vi "UI - Main UI config.vi"() -> ()   [LabVIEW 2020, in "Configuration.lvclass"]
doc: "Module UI that appears in the Configuration UI.\n____\nPeloton Config 2.0.0.9\nCopyright (c) 2024, Peloton"
uses:
  Configuration.lvclass
  <vilib>/Peloton/Peloton Config/DCFG Framework/Init UI Params--cluster.ctl
  <vilib>/Peloton/Peloton Config/DCFG Framework/Configuration_class/Configuration.lvclass
  <vilib>/Peloton/Peloton Config/DCFG Framework/Stop Argument--cluster.ctl
  <vilib>/Peloton/Peloton Config/DCFG Framework/Send Config to Page Argument--cluster.ctl
  <vilib>/Peloton/Peloton Config/DCFG Framework/Send Stop to Page Argument--cluster.ctl
  C:/Program Files (x86)/National Instruments/LabVIEW 2020/vi.lib/Peloton/Peloton Config/DCFG Framework/Configuration_class/Configuration.lvclass
  <vilib>/Peloton/Peloton Config/DCFG Framework/Configuration_class/Configuration.lvclass/Configuration.ctl
  Configuration--cluster.ctl
  Configuration.lvclass/Configuration.ctl
  Set Configuration.vi
  Get Configuration.vi
  <vilib>/Peloton/Peloton Config/DCFG Framework/Configuration_class/Get Name.vi
  <vilib>/Peloton/Peloton Config/DCFG Framework/Peloton_lib_DCFG Framework.lvlib
panel:
  in  "B":dbl
  in  "a":dbl
  in  "Init UI Params":T1
  # "Define the Default Configuration UI here."
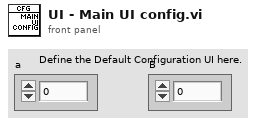
[diagram p1: front panel]
types:
  T1 = typedef "Peloton_lib_DCFG Framework.lvlib/Init UI Params--cluster.ctl" = cluster{"Initial Config":refnum<class "Configuration.lvclass">, "Stop CFG Module":refnum<user-event>, "Send Config to Page":refnum<user-event>, "Send Stop to Page":refnum<user-event>, "Reset Page Defaults":refnum<user-event>}
  T2 = enum32{"Invalid", "Standard", "Closed", "Hidden", "Minimized", "Maximized"}
  T3 = typedef "Configuration.lvclass/Configuration--cluster.ctl" = cluster{"a":dbl, "B":dbl}
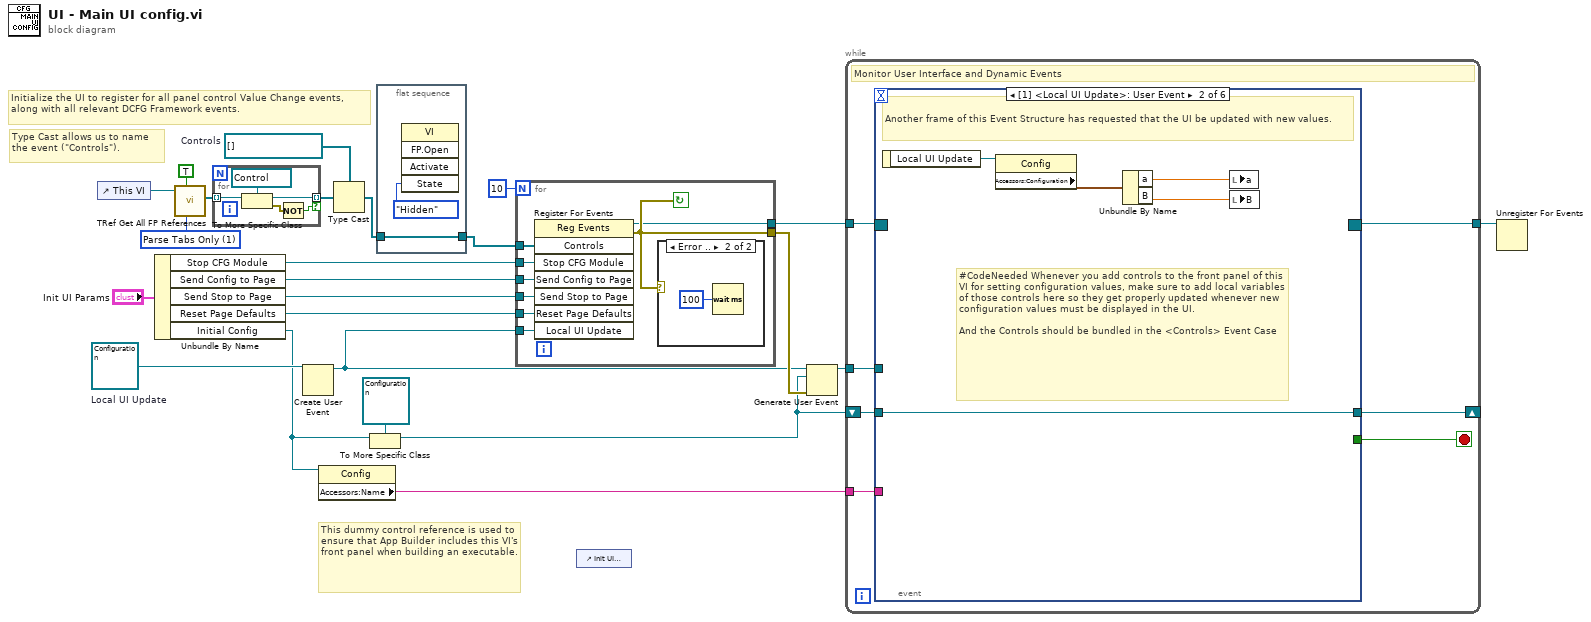
[diagram p0: block diagram]
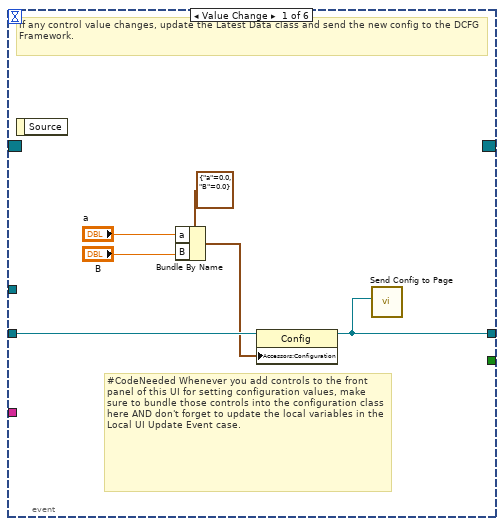
[diagram p3: hidden frame]
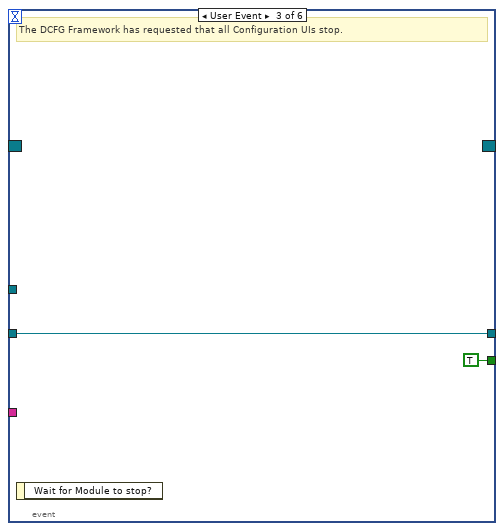
[diagram p4: hidden frame]
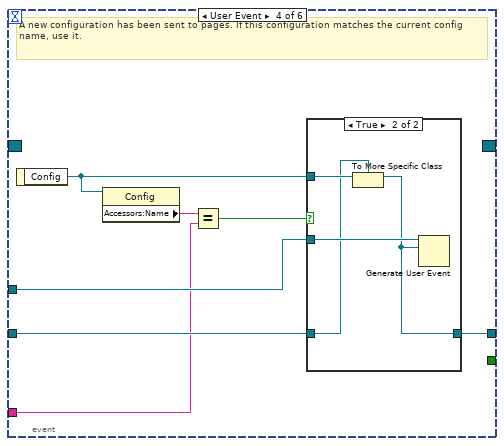
[diagram p5: hidden frame]
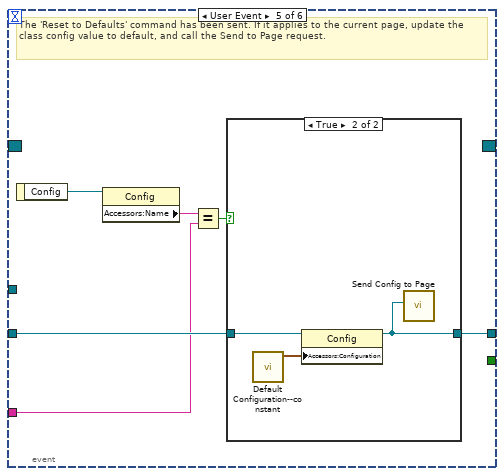
[diagram p7: hidden frame]
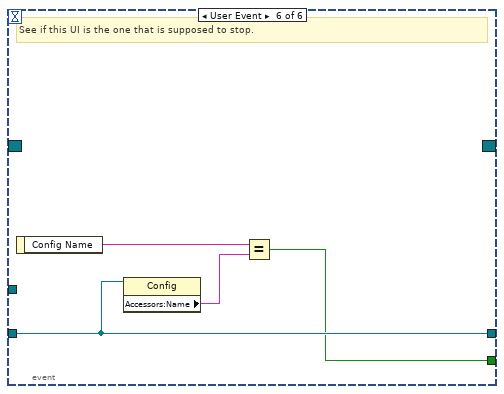
[diagram p9: hidden frame]
diagram:
  w6 = refnum<vi>[] []  # Controls
  w11 = u16 1 items=["Parse All", "Parse Tabs Only"] ("Parsing Rule")
  w21 = refnum<class "Configuration.lvclass"> refnum  # Local UI Update
  # "Type Cast allows us to name the event (\"Controls\")."
  # "Initialize the UI to register for all panel control Value Change events, along with all relevant DCFG Framework events."
  # "This dummy control reference is used to ensure that App Builder includes this VI's front panel when building an executable."
  n1 = control-ref of="This VI"() -> (w1:refnum<vi>)
  n2 = Unbundle By Name("Init UI Params") -> ("Stop CFG Module"=w18:refnum<user-event>, "Send Config to Page"=w17:refnum<user-event>, "Send Stop to Page"=w16:refnum<user-event>, "Reset Page Defaults"=w15:refnum<user-event>, "Initial Config"=w8:refnum<class "Configuration.lvclass">)
  n3 = call <vilib>:"TRef Get All FP References.vi"("Parsing Rule"=w11, "Ignore Decorations?"=TRUE, "VI Refnum"=w1) -> ("All FP Objects"=w12:refnum<vi>[])  [unwired: 4 in, 4 out]
  n4 = for {
    tunnel: w12 -> [w28] mode=indexing
    tunnel: [w27] -> w5 mode=indexing if=w25
    n5 = To More Specific Class(target class=refnum<vi> refnum ("Controls"), reference=w28) -> (specific class reference=w27:refnum<vi>, error out=w29:errorcluster)  [unwired: 1 in]
    n6 = Not(x=w29) -> (.not. x?=w25:bool)
  }
  n7 = Create User Event(user event datatype=w21) -> (user event=w14:refnum<user-event>)  [unwired: 1 in, 1 out]
  n8 = property class="Config"(reference=w8) -> ("Accessors:Name"=w7:string)  [unwired: 1 in, 2 out]
  n9 = Type Cast(type=w6, x=w5) -> (*(type *) &x=w4:refnum<vi>[])
  n10 = To More Specific Class(target class=refnum<class "Configuration.lvclass"> refnum ("Sample Module 1.lvlib:Config"), reference=w8) -> (specific class reference=w10:refnum<class "Configuration.lvclass">)  [unwired: 1 in, 1 out]
  n11 = flat-sequence {
    tunnel: w4 -> [w31]
    tunnel: [w31] -> w3
    frame #0 {
      n12 = invoke on="Invoke Node" class="VI" method="FP.Open"("State"=T2."Hidden") -> ()  [unwired: 4 in, 5 out]
    }
  }
  n13 = for {
    N: 10 -> [_]
    tunnel: [w38] -> w23
    tunnel: [w39] -> w24
    tunnel: w18 -> [w37]
    tunnel: w17 -> [w36]
    tunnel: w16 -> [w35]
    tunnel: w15 -> [w34]
    tunnel: w14 -> [w33]
    tunnel: w3 -> [w32]
    stop <- w39 continue-if-true
    n14 = register-events(w32, w37, w36, w35, w34, w33) -> (reference out=w38:refnum<event-registration>, error out=w39:errorcluster)  [unwired: 2 in]
    n15 = case shown="Error .." w39 {
      frame No Error {
      }
      frame Error {
        n16 = Wait (ms)(milliseconds to wait=u32 100) -> ()  [unwired: 1 out]
      }
    }
  }
  n17 = control-ref of="Init UI Params"() -> ()  [unwired: 1 out]
  n18 = Generate User Event(user event=w14, event data cluster=w10, error in=w24) -> (user event out=w20:refnum<user-event>)  [unwired: 1 in, 1 out]
  n19 = while {
    tunnel: w23 -> [w47]
    tunnel: [w46] -> w22
    shift-right: [w42] -> _
    shift-left: w10 -> [w45]
    tunnel: w20 -> [w43]
    tunnel: w7 -> [w41]
    stop <- w44 stop-if-true
    # "Monitor User Interface and Dynamic Events"
    n20 = event shown="[1] <Local UI Update>: User Event" {
      selector: w47 -> [_ _ _ _ _ _]
      dyn-events: [_ _ _ _ _ _] -> w46
      timeout: _ -> [_ _ _ _ _ _]
      tunnel: w45 -> [w52 w58 w60 w65 w77 w86]
      tunnel: [w51 w58 w60 w66 w78 w86] -> w42
      tunnel: [_ _ TRUE ("Addressed to this instance?") _ _ w83] -> w44
      tunnel: w43 -> [_ _ _ w67 _ _]
      tunnel: w41 -> [_ _ _ w62 w74 _]
      event Value Change {
        # "#CodeNeeded Whenever you add controls to the front panel of this UI for setting configuration values, make sure to bundle those controls into the configuration class here AND don't forget to update the local variables in the Local UI Update Event case."
        # "If any control value changes, update the Latest Data class and send the new config to the DCFG Framework."
        n21 = event-data() -> ()  [unwired: 1 in, 1 out]
        n22 = Bundle By Name(cluster=T3 {"a"=0.0, "B"=0.0} ("Configuration"), "a"="a", "B"="B") -> (w50:T3)
        n23 = property class="Config"(reference=w52, "Accessors:Configuration"=w50) -> (reference out=w51:refnum<class "Configuration.lvclass">)  [unwired: 1 in, 1 out]
        n24 = call <vilib>:"Send Config to Page.vi"("Config"=w51) -> ()  [unwired: 10 in, 1 out]
      }
      event User Event {
        # "#CodeNeeded Whenever you add controls to the front panel of this VI for setting configuration values, make sure to add local variables of those controls here so they get properly updated whenever new configuration values must be displayed in the UI.\n\nAnd the Controls should be bundled in the <Controls> Event Case"
        # "Another frame of this Event Structure has requested that the UI be updated with new values."
        n25 = event-data() -> ("Local UI Update"=w57:refnum<class "Configuration.lvclass">)  [unwired: 1 in]
        n26 = property class="Config"(reference=w57) -> ("Accessors:Configuration"=w56:T3)  [unwired: 1 in, 2 out]
        n27 = Unbundle By Name(w56) -> ("a"=w55:dbl, "B"=w54:dbl)
        n28 = local write "a"(w55) -> ()
        n29 = local write "B"(w54) -> ()
      }
      event User Event {
        # "The DCFG Framework has requested that all Configuration UIs stop."
        n30 = event-data() -> ()  [unwired: 1 in, 1 out]
      }
      event User Event {
        # "A new configuration has been sent to pages. If this configuration matches the current config name, use it."
        n31 = event-data() -> ("Config"=w64:refnum<class "Configuration.lvclass">)  [unwired: 1 in]
        n32 = property class="Config"(reference=w64) -> ("Accessors:Name"=w63:string)  [unwired: 1 in, 2 out]
        n33 = Equal?(x=w63, y=w62) -> (x = y?=w61:bool)
        n34 = case shown="True" w61 {
          tunnel: w67 -> [_ w72]
          tunnel: w65 -> [w68 w69]
          tunnel: [w68 w71] -> w66
          tunnel: w64 -> [_ w70]
          frame False {
          }
          frame True {
            n35 = To More Specific Class(target class=w69, reference=w70) -> (specific class reference=w71:refnum<class "Configuration.lvclass">)  [unwired: 1 in, 1 out]
            n36 = Generate User Event(user event=w72, event data cluster=w71) -> ()  [unwired: 2 in, 2 out]
          }
        }
      }
      event User Event {
        # "The 'Reset to Defaults' command has been sent. If it applies to the current page, update the class config value to default, and call the Send to Page request."
        n37 = event-data() -> ("Config"=w76:refnum<class "Configuration.lvclass">)  [unwired: 1 in]
        n38 = property class="Config"(reference=w76) -> ("Accessors:Name"=w75:string)  [unwired: 1 in, 2 out]
        n39 = Equal?(x=w75, y=w74) -> (x = y?=w73:bool)
        n40 = case shown="True" w73 {
          tunnel: w77 -> [w79 w82]
          tunnel: [w79 w80] -> w78
          frame False {
          }
          frame True {
            n41 = call "Default Configuration--constant.vi"() -> ("Default Configuration"=w81:T3)  [unwired: 11 in]
            n42 = property class="Config"(reference=w82, "Accessors:Configuration"=w81) -> (reference out=w80:refnum<class "Configuration.lvclass">)  [unwired: 1 in, 1 out]
            n43 = call <vilib>:"Send Config to Page.vi"("Config"=w80) -> ()  [unwired: 10 in, 1 out]
          }
        }
      }
      event User Event {
        # "See if this UI is the one that is supposed to stop."
        n44 = event-data() -> ("Config Name"=w85:string)  [unwired: 1 in]
        n45 = property class="Config"(reference=w86) -> ("Accessors:Name"=w84:string)  [unwired: 1 in, 2 out]
        n46 = Equal?(x=w85, y=w84) -> (x = y?=w83:bool)
      }
    }
  }
  n47 = Unregister For Events(event registration refnum=w22) -> ()  [unwired: 1 in, 1 out]
